vi "Ej 5 Variables Locales.vi"() -> ()   [LabVIEW 2021]
panel:
  out "Waveform Chart 2":dbl(graph)
  out "Waveform Chart":dbl(graph)
  in  "Boolean":bool
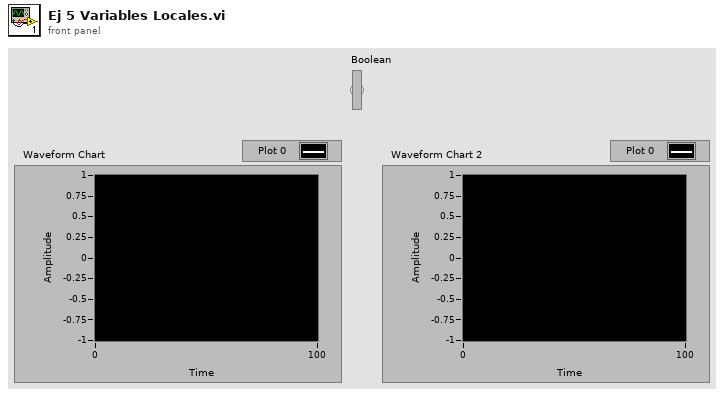
[diagram p1: front panel]
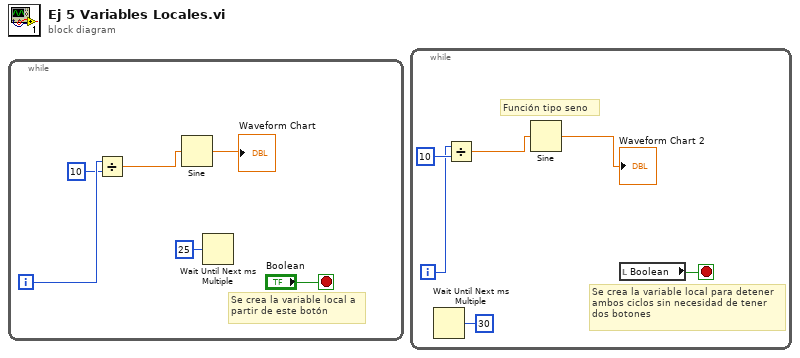
[diagram p0: block diagram]
diagram:
  n1 = while {
    i -> [w5]
    stop <- "Boolean" stop-if-true
    # "Se crea la variable local a \npartir de este botón"
    n2 = Divide(x=w5, y=10) -> (x/y=w6:dbl)
    n3 = Sine(x=w6) -> (sin(x)=→"Waveform Chart":dbl)
    n4 = Wait Until Next ms Multiple(millisecond multiple=u32 25) -> ()  [unwired: 1 out]
  }
  n5 = while {
    i -> [w10]
    stop <- w7 stop-if-true
    # "Función tipo seno"
    # "Se crea la variable local para detener\nambos ciclos sin necesidad de tener \ndos botones"
    n6 = Wait Until Next ms Multiple(millisecond multiple=u32 30) -> ()  [unwired: 1 out]
    n7 = Divide(x=w10, y=10) -> (x/y=w12:dbl)
    n8 = Sine(x=w12) -> (sin(x)=→"Waveform Chart 2":dbl)
    n9 = local read "Boolean"() -> (w7:bool)
  }
